vi "meta range at.vi"(8 "error in (no error)":errorcluster, 9 "range_out":cluster{"start":dbl, "stop":dbl, "step":dbl}, 10 "num":u64, 11 "h":u64) -> (0 "error out":errorcluster, 1 "range_out out":cluster{"start":dbl, "stop":dbl, "step":dbl}, 3 "function return":u32(ring))   [LabVIEW 2023, in "uhd.lvlib"]
doc: "UHD_API uhd_error uhd_meta_range_at(\n uhd_meta_range_handle h, size_t num, uhd_range_t* range_out);"
uses:
  <userlib>/uhd/uhd.lvlib
  <userlib>/uhd/uhd.dll
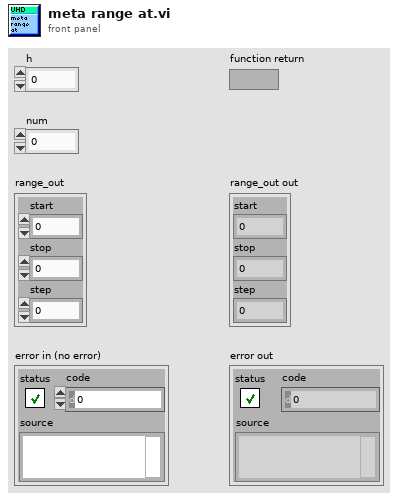
[diagram p1: front panel]
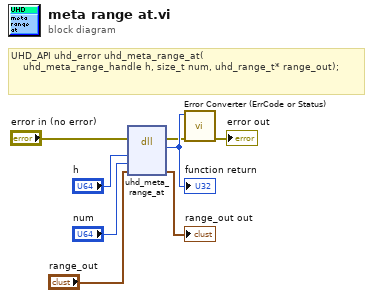
[diagram p0: block diagram]
diagram:
  # "UHD_API uhd_error uhd_meta_range_at(\n    uhd_meta_range_handle h, size_t num, uhd_range_t* range_out);"
  n1 = dll-call lib="C:/Program Files/National Instruments/LabVIEW 2023/user.lib/uhd/uhd.*" fn="uhd_meta_range_at"(error in="error in (no error)", "h"="h", "num"="num", "range_out"="range_out") -> (error out=w2:errorcluster, w8:u32, "range_out"=→"range_out out":cluster{"start":dbl, "stop":dbl, "step":dbl})  [unwired: 4 in, 1 out]
  "function return" <- w8
  n2 = call <userlib>:"Error Converter (ErrCode or Status).vi"("error in (no error)"=w2, "error code"=w8) -> ("error out"=→"error out":errorcluster)  [unwired: 9 in]
